vi "Get Arm Source Name.vi"(8 "error in (no error)":errorcluster {"code" format="%.0x"}, 9 "SourceNameBufferSize":i32=256 caption="SourceNameBufferSize (256)", 10 "SourceIndex":i32=1 caption="SourceIndex (1)" format="%.0g", 11 "instrument handle":refnum<k15>) -> (0 "error out":errorcluster {"code" format="%.0x"}, 2 "SourceName":string, 3 "instrument handle out":refnum<k15>)   [LabVIEW 2009, in "Keysight XSAn.lvlib"]
doc: "This VI returns the physical repeated capability identifier that corresponds to the one-based index that the user specifies. If the value that the user passes for the SourceIndex parameter is less than one or greater than the value of the Arm Source Count property, the VI returns an empty string in the SourceName parameter and returns an error. For custom arm sources added vith the Add Arm Source function, this function returns the arm source name in the original casing used when Add Arm Source was called.\n\nSupported Models: All supported"
uses:
  <instrlib>/Keysight XSAn/Keysight XSAn.lvlib
  AgXSAn.dll
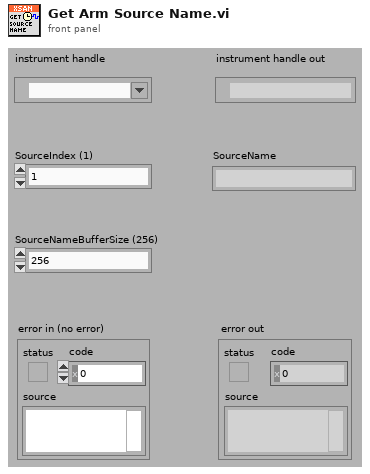
[diagram p1: front panel]
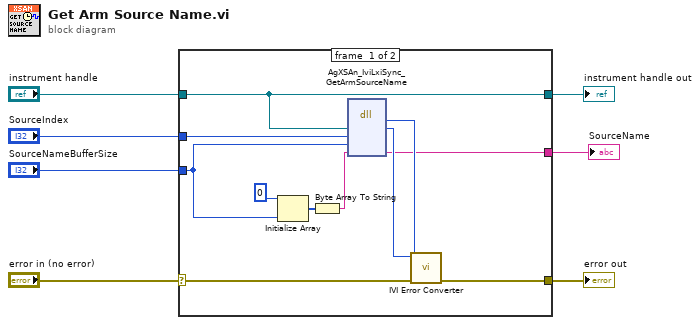
[diagram p0: block diagram]
diagram:
  n1 = case shown="No Error" "error in (no error)" {
    selector: "error in (no error)" -> [w16 w20]
    tunnel: [w15 w20] -> w7
    tunnel: "instrument handle" -> [w9 w19]
    tunnel: "SourceIndex" -> [w14 _]
    tunnel: "SourceNameBufferSize" -> [w8 _]
    tunnel: [w10 _] -> w2
    tunnel: [w9 w19] -> w1
    frame #0 {
      n2 = Initialize Array(u8 0 ("element"), w8) -> (w12:u8[])
      n3 = Byte Array To String(unsigned byte array=w12) -> (string=w13:string)
      n4 = dll-call lib="AgXSAn**.dll" fn="AgXSAn_IviLxiSync_GetArmSourceName"("Vi"=w9, "SourceIndex"=w14, "SourceNameBufferSize"=w8, "SourceName"=w13) -> (w17:i32, "Vi"=w18:u32, "SourceName"=w10:string)  [unwired: 5 in, 2 out]
      n5 = call <instrlib>:"IVI Error Converter.vi"("error in (no error)"=w16, "IVI error code (0)"=w17, "instrument handle"=w18) -> ("error out"=w15:errorcluster)  [unwired: 7 in, 1 out]
    }
    frame #1 {
    }
  }
  "error out" <- w7
  "instrument handle out" <- w1
  "SourceName" <- w2
